vi "Set Cursor Busy State.vi"(8 "Error In":errorcluster, 10 "Busy?":bool, 11 "Splitter Settings UI in":refnum<class "Splitter Settings UI.lvclass">) -> (0 "Error Out":errorcluster, 3 "Splitter Settings UI out":refnum<class "Splitter Settings UI.lvclass">)   [LabVIEW 2019, in "Splitter Settings UI.lvlib" / "Splitter Settings UI.lvclass"]
uses:
  <resource>/dialog/QuickDrop/plugins/PaneRelief/Classes/Splitter Settings UI/Splitter Settings UI/Splitter Settings UI.lvclass
  <vilib>/MGI/Panel Manager/Panel Actor/Panel Actor/Panel Actor.lvclass
  <vilib>/MGI/Panel Manager/Panel/Cursor/Cursor.lvclass
  C:/Program Files (x86)/National Instruments/LabVIEW 2019/vi.lib/MGI/Panel Manager/Panel Actor/Panel Actor/Panel Actor.lvclass
  C:/Program Files (x86)/National Instruments/LabVIEW 2019/vi.lib/MGI/Monitored Actor/Monitored Actor/Monitored Actor/Monitored Actor.lvclass
  C:/Program Files (x86)/National Instruments/LabVIEW 2019/vi.lib/ActorFramework/Actor/Actor.lvclass
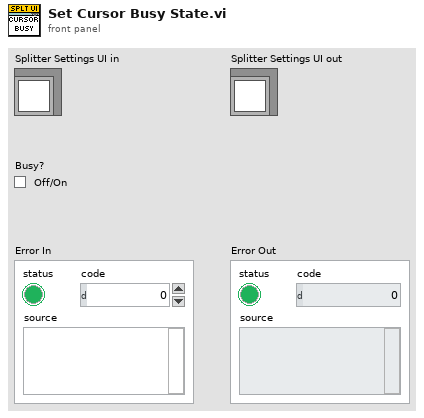
[diagram p1: front panel]
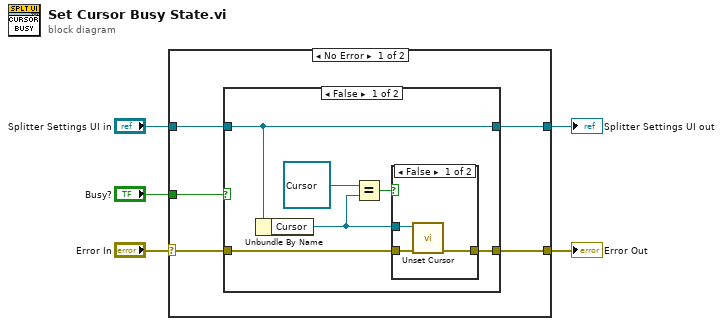
[diagram p0: block diagram]
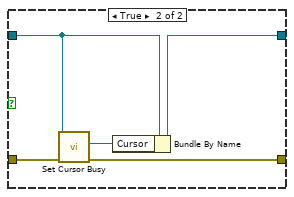
[diagram p3: hidden frame]
diagram:
  n1 = case shown="No Error" "Error In" {
    selector: "Error In" -> [w10 w27]
    tunnel: [w9 w27] -> w2
    tunnel: [w8 w26] -> w4
    tunnel: "Splitter Settings UI in" -> [w7 w26]
    tunnel: "Busy?" -> [w6 _]
    frame No Error {
      n2 = case shown="False" w6 {
        tunnel: w10 -> [w16 w25]
        tunnel: [w15 w24] -> w9
        tunnel: [w14 w23] -> w8
        tunnel: w7 -> [w14 w22]
        frame False {
          n3 = Unbundle By Name(w14) -> ("Cursor"=w12:refnum<class "Cursor.lvclass">)
          n4 = Equal?(x=refnum<class "Cursor.lvclass"> refnum ("Cursor"), y=w12) -> (x = y?=w11:bool)
          n5 = case shown="False" w11 {
            tunnel: w16 -> [w19 w20]
            tunnel: [w18 w20] -> w15
            tunnel: w12 -> [w17 _]
            frame False {
              n6 = call <vilib>:"Unset Cursor.vi"("error in (no error)"=w19, "Cursor in"=w17) -> ("error out"=w18:errorcluster)  [unwired: 9 in]
            }
            frame True {
            }
          }
        }
        frame True {
          n7 = call <vilib>:"Set Cursor Busy.vi"("error in (no error)"=w25, "Panel Actor in"=w22) -> ("error out"=w24:errorcluster, "Cursor"=w21:refnum<class "Cursor.lvclass">)  [unwired: 8 in]
          n8 = Bundle By Name(cluster=w22, "Cursor"=w21) -> (w23:refnum<class "Splitter Settings UI.lvclass">)
        }
      }
    }
    frame Error {
    }
  }
  "Splitter Settings UI out" <- w4
  "Error Out" <- w2
